vi "Read - NI.vi"(8 "error in (no error)":errorcluster, 10 "Maximum Time (msec)":i32=-1, 11 "instrument handle":refnum<k15>) -> (0 "error out":errorcluster, 2 "Measurement":dbl format="%.5f", 3 "instrument handle out":refnum<k15>)   [LabVIEW 2020]
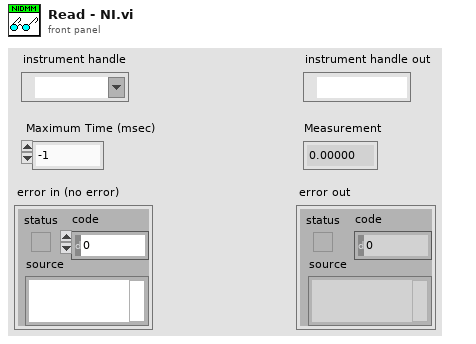
[diagram p1: front panel]
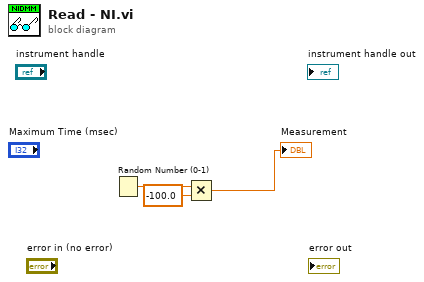
[diagram p0: block diagram]
diagram:
  n1 = Random Number (0-1)() -> (number: 0 to 1=w3:dbl)
  n2 = Multiply(x=w3, y=-100.0) -> (x*y=→"Measurement":dbl)
